vi "Query with 2D Integer Result.vi"(8 "error in (no error)":errorcluster, 10 "Query string":string, 11 "mysql in":refnum<class "mysql.lvclass">) -> (0 "error out":errorcluster, 2 "Result":i32[][](array[numeric]), 3 "mysql out":refnum<class "mysql.lvclass">)   [LabVIEW 2020, in "mysql.lvlib" / "mysql.lvclass"]
uses:
  mysql.lvclass
  c1dd671d-7da9-498e-8da8-d643cc8ab19e.vi
  c1dd671d-7da9-498e-8da8-d643cc8ab19e.vi/4a45eab4-823c-4b0d-b546-ca70823bf7fb.vi
  c1dd671d-7da9-498e-8da8-d643cc8ab19e.vi/412fbfd5-24cf-4923-9758-af6966e55a83.vi
  private/Mysql command.vi
  private/Mysql data reader 2D integer.vi
  private/ping connection and reopen if needed.vi
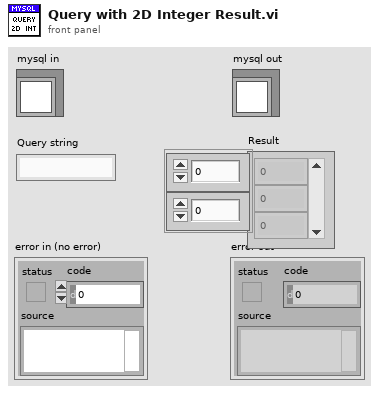
[diagram p1: front panel]
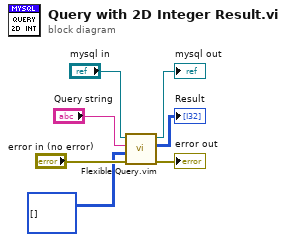
[diagram p0: block diagram]
diagram:
  n1 = call "Flexible Query.vim"("error in (no error)"="error in (no error)", "Type in"=i32[][] [] ("Result 2"), "Query string"="Query string", "mysql in"="mysql in") -> ("error out"=→"error out":errorcluster, "Result"=→"Result":i32[][], "mysql out"=→"mysql out":refnum<class "mysql.lvclass">)  [unwired: 5 in]
